vi "RunScript.vi"(8 "error in":errorcluster, 10 "script":string, 11 "VISA Refnum in":refnum<visa-resource-name>) -> (0 "error out":errorcluster, 2 "Tx":string, 3 "VISA Refnum out":refnum<visa-resource-name>)   [LabVIEW 2017]
panel:
  out "Reply":string
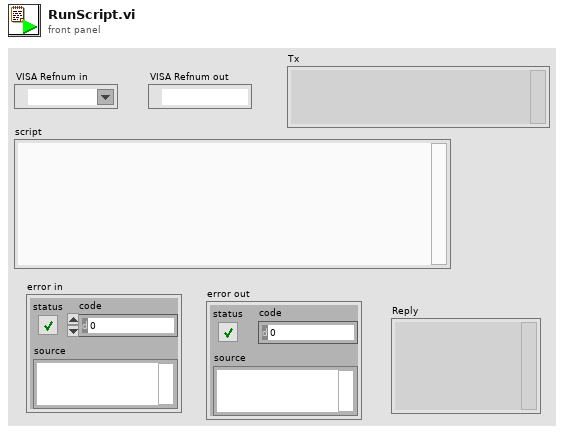
[diagram p1: front panel]
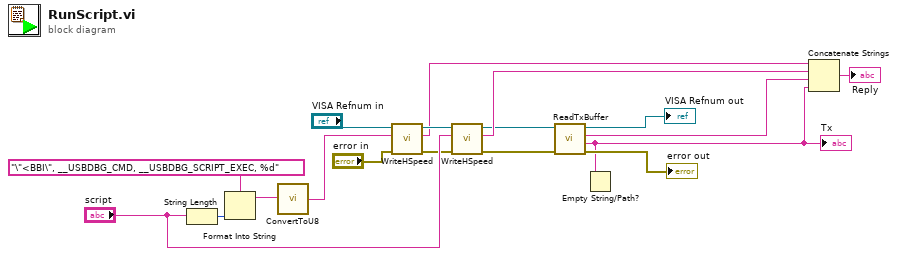
[diagram p0: block diagram]
diagram:
  n1 = String Length(string="script") -> (length=w17:i32)
  n2 = Format Into String(format string="\"<BBI\", __USBDBG_CMD, __USBDBG_SCRIPT_EXEC, %d" ("write buffer"), w17) -> (resulting string=w4:string)  [unwired: 2 in, 1 out]
  n3 = call <userlib>:"ConvertToU8.vi"("struct"=w4) -> ("Binary"=w3:string)
  n4 = call <userlib>:"WriteHSpeed.vi"("error in"="error in", "write buffer"=w3, "VISA Refnum in"="VISA Refnum in") -> ("error out"=w12:errorcluster, "read buffer"=w10:string, "VISA Refnum out"=w15:refnum<visa-resource-name>)  [unwired: 6 in]
  n5 = call <userlib>:"WriteHSpeed.vi"("error in"=w12, "write buffer"="script", "VISA Refnum in"=w15) -> ("error out"=w1:errorcluster, "read buffer"=w11:string, "VISA Refnum out"=w8:refnum<visa-resource-name>)  [unwired: 6 in]
  n6 = call <userlib>:"ReadTxBuffer.vi"("error in"=w1, "VISA Refnum in"=w8) -> ("error out"=→"error out":errorcluster, "Tx Buffer"=w2:string, "Tx Buffer Len"=w7:string, "VISA Refnum out"=→"VISA Refnum out":refnum<visa-resource-name>)  [unwired: 6 in]
  "Tx" <- w2
  n7 = Empty String/Path?(string/path=w2) -> ()  [unwired: 1 out]
  n8 = Concatenate Strings(w10, w11, w7, w2) -> (→"Reply":string)
